vi "Write Return VF Setpoint Msg.vi"(10 "Return VF Setpoint Msg":refnum<class "Return VF Setpoint Msg.lvclass">, 11 "Optimization in":refnum<class "Optimization.lvclass">) -> (3 "Optimization out":refnum<class "Optimization.lvclass">)   [LabVIEW 2016, in "Optimization Framework.lvlib" / "Optimization.lvclass"]
uses:
  Optimization.lvclass
  Optimization Messages/Return VF Setpoint Msg/Return VF Setpoint Msg.lvclass
  Optimization.lvclass/Optimization.ctl
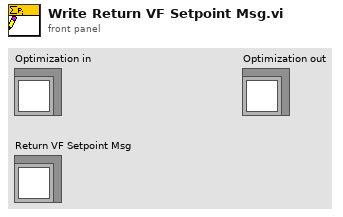
[diagram p1: front panel]
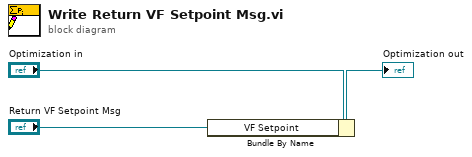
[diagram p0: block diagram]
diagram:
  n1 = Bundle By Name(cluster="Optimization in", "VF Setpoint"="Return VF Setpoint Msg") -> (→"Optimization out":refnum<class "Optimization.lvclass">)
